vi "DataToDataBase.vi"(10 "Poperties":T2, 11 "RawData":dbl[][](array[numeric])) -> (3 "DataToDataBase":T1)   [LabVIEW 2019]
uses:
  Communication/TypeDef/#TypeDef_PropertiesToSave.ctl
  TypeDef/#TypeDef_DataToDatabase.ctl
  Global_Freq.vi
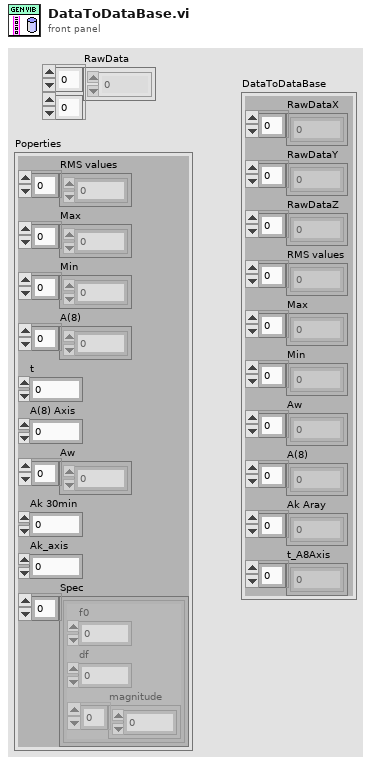
[diagram p1: front panel]
types:
  T1 = typedef "#TypeDef_DataToDatabase.ctl" = cluster{"RawDataX":dbl[], "RawDataY":dbl[], "RawDataZ":dbl[], "RMS values":dbl[], "Max":dbl[], "Min":dbl[], "Aw":dbl[], "A(8)":dbl[], "Ak Aray":dbl[], "t_A8Axis":dbl[]}
  T2 = typedef "#TypeDef_PropertiesToSave.ctl" = cluster{"RMS values":dbl[], "Max":dbl[], "Min":dbl[], "A(8)":dbl[], "t":dbl, "A(8) Axis":dbl, "Aw":dbl[], "Ak 30min":dbl, "Ak_axis":i32, "Spec":cluster{"f0":dbl, "df":dbl, "magnitude":dbl[]}[]}
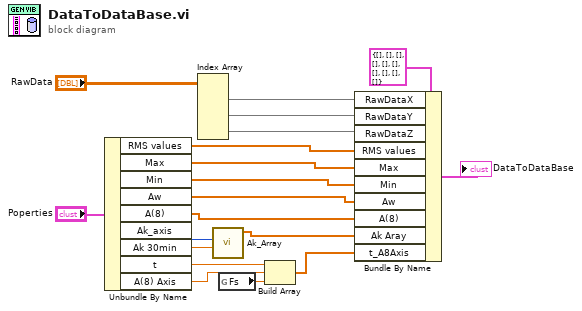
[diagram p0: block diagram]
diagram:
  n1 = Unbundle By Name("Poperties") -> ("RMS values"=w2:dbl[], "Max"=w3:dbl[], "Min"=w4:dbl[], "Aw"=w5:dbl[], "A(8)"=w6:dbl[], "Ak_axis"=w14:i32, "Ak 30min"=w15:dbl, "t"=w7:dbl, "A(8) Axis"=w8:dbl)
  n2 = Index Array(array="RawData") -> (element #1=w11:dbl[], element #2=w12:dbl[], element #3=w13:dbl[])  [unwired: 6 in]
  n3 = call "Ak_Array.vi"("Ak 30min"=w15, "Ak_axis"=w14) -> ("Ak Aray"=w16:dbl[])  [unwired: 9 in]
  n4 = global read "Global_Freq.vi" "Fs"() -> (w1:dbl)
  n5 = Build Array(w7, w8, w1) -> (w9:dbl[])
  n6 = Bundle By Name(cluster=T1 {"RawDataX"=[], "RawDataY"=[], "RawDataZ"=[], "RMS values"=[], "Max"=[], "Min"=[], "Aw"=[], "A(8)"=[], "Ak Aray"=[], "t_A8Axis"=[]} ("DataToDataBase"), "RawDataX"=w11, "RawDataY"=w12, "RawDataZ"=w13, "RMS values"=w2, "Max"=w3, "Min"=w4, "Aw"=w5, "A(8)"=w6, "Ak Aray"=w16, "t_A8Axis"=w9) -> (→"DataToDataBase":T1)
